vi "New Channel from Term Info.vi"(1 "Channel Settings ducktype":T4={"Name"="sim1", "Terminal Information"={"IO Device"=enum."none", "Channel"=0, "Sensor Type"=enum."Voltage"}}) -> (0 "New Channel":T1={"Name"="", "Terminal Information"={"IO Device"=enum."none", "Channel"=0, "Sensor Type"=enum."Voltage"}, "Calibration Information"={"Excitation Voltage"=1.0, "Calibration Factor"=1.0, "Zero Value"=0.0, "Calibration Formula"="(x-x0) / (Ve * CF)", "Units"="V"}})   [LabVIEW 2021, in "Acquisition.lvlib"]
doc: "Return a new instance of 'Channel Settings' using the name and terminal information from 'Channel Settings ducktype'."
uses:
  Acquisition.lvlib
  IO Device.ctl
  Sensor Type.ctl
  Channel Settings.ctl
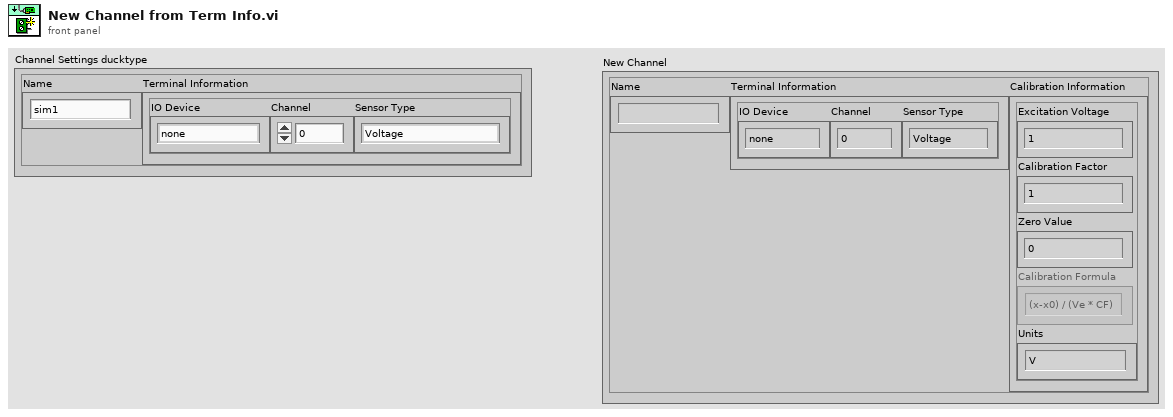
[diagram p1: front panel]
types:
  T1 = typedef "Acquisition.lvlib/Channel Settings.ctl" = cluster{"Name":string, "Terminal Information":cluster{"IO Device":T2, "Channel":i32, "Sensor Type":T3}, "Calibration Information":cluster{"Excitation Voltage":dbl, "Calibration Factor":dbl, "Zero Value":dbl, "Calibration Formula":string, "Units":string}}
  T2 = typedef "Acquisition.lvlib/IO Device.ctl" = enum16{"none", "9219", "9401"}
  T3 = typedef "Acquisition.lvlib/Sensor Type.ctl" = enum16{"Voltage", "Load", "Pressure", "Encoder"}
  T4 = cluster{"Name":string, "Terminal Information":cluster{"IO Device":T2, "Channel":i32, "Sensor Type":T3}}
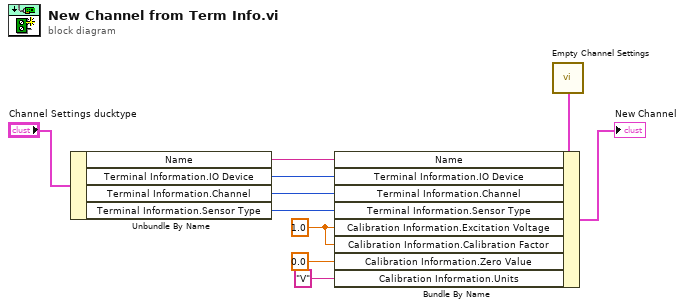
[diagram p0: block diagram]
diagram:
  w3 = 1.0 ("Calibration Information.Excitation Voltage")
  n1 = Unbundle By Name("Channel Settings ducktype") -> ("Name"=w7:string, "Terminal Information.IO Device"=w6:T2, "Terminal Information.Channel"=w5:i32, "Terminal Information.Sensor Type"=w4:T3)
  n2 = call "Empty Channel Settings.vi"() -> ("Channel Settings"=w10:T1)
  n3 = Bundle By Name(cluster=w10, "Name"=w7, "Terminal Information.IO Device"=w6, "Terminal Information.Channel"=w5, "Terminal Information.Sensor Type"=w4, "Calibration Information.Excitation Voltage"=w3, "Calibration Information.Calibration Factor"=w3, "Calibration Information.Zero Value"=0.0, "Calibration Information.Units"="V") -> (→"New Channel":T1)
